vi "Search_1D_Array(STR).vi"(0 "Array - String":string[](array[string]), 2 "Element Data":string, 3 "Start Index (0)":i32) -> (7 "Indicies of Elements":i32[](array[numeric]), 9 "Array of Elements":string[](array[string]))   [LabVIEW 2011]
doc: "Searches for all element data matches in array"
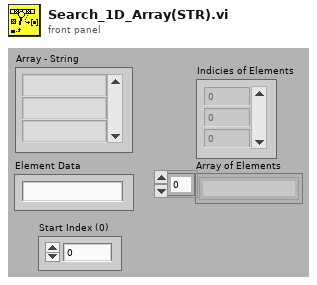
[diagram p1: front panel]
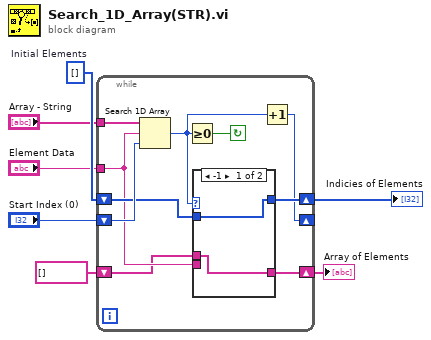
[diagram p0: block diagram]
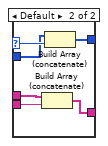
[diagram p2: hidden frame]
diagram:
  w7 = i32[] []  # Initial Elements
  n1 = while {
    shift-right: [w11] -> _
    shift-left: "Start Index (0)" -> [w17]
    shift-right: [w14] -> w3
    shift-left: w7 -> [w15]
    tunnel: "Array - String" -> [w16]
    tunnel: "Element Data" -> [w10]
    shift-right: [w9] -> w1
    shift-left: string[] [] -> [w8]
    stop <- w12 continue-if-true
    n2 = Search 1D Array(1D array=w16, element=w10, start index (0)=w17) -> (index of element=w13:i32)
    n3 = Greater Or Equal To 0?(x=w13) -> (x >= 0?=w12:bool)
    n4 = case shown="-1" w13 {
      selector: w13 -> [_ w25]
      tunnel: w15 -> [w19 w24]
      tunnel: [w19 w23] -> w14
      tunnel: w10 -> [_ w22]
      tunnel: [w18 w21] -> w9
      tunnel: w8 -> [w18 w20]
      frame -1 {
      }
      frame Default {
        n5 = Build Array (concatenate)(w20, w22) -> (w21:string[])
        n6 = Build Array (concatenate)(w24, w25) -> (w23:i32[])
      }
    }
    n7 = Increment(x=w13) -> (x+1=w11:i32)
  }
  "Indicies of Elements" <- w3
  "Array of Elements" <- w1
